vi "CameraServoPWM.vi"(11 "Position":i32) -> ()   [LabVIEW 2018]
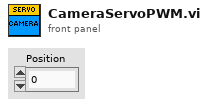
[diagram p1: front panel]
types:
  T1 = typedef "WPI_PWMDeviceRef.ctl" = cluster{"DeviceStatus":errorcluster, "PWM Channel":T2}
  T2 = typedef "FPGA_DIOPWMChannel.ctl" = enum8{"PWM 0", "PWM 1", "PWM 2", "PWM 3", "PWM 4", "PWM 5", "PWM 6", "PWM 7", "PWM 8", "PWM 9", "PWM MXP 0", "PWM MXP 1", "PWM MXP 2", "PWM MXP 3", "PWM MXP 4", "PWM MXP 5", "PWM MXP 6", "PWM MXP 7", "PWM MXP 8", "PWM MXP 9", "Invalid"}
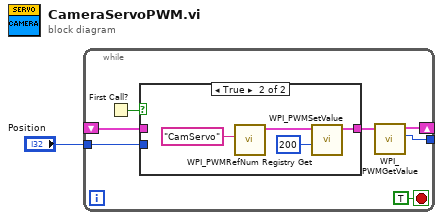
[diagram p0: block diagram]
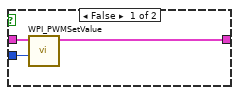
[diagram p2: hidden frame]
diagram:
  n1 = while {
    tunnel: "Position" -> [w8]
    shift-right: [w4] -> _
    shift-left: _ -> [w7]
    tunnel: [w3] -> _
    stop <- TRUE stop-if-true
    n2 = First Call?() -> (First Call?: T/F=w5:bool)
    n3 = case shown="True" w5 {
      tunnel: w8 -> [w10 _]
      tunnel: [w11 w12] -> w2
      tunnel: w7 -> [w9 _]
      frame False {
        n4 = call <vilib>:"WPI_PWMSetValue.vi"("Value"=w10, "PWMDeviceRef"=w9) -> ("PWMDeviceRef"=w11:T1)  [unwired: 8 in, 1 out]
      }
      frame True {
        n5 = call <vilib>:"WPI_PWMRefNum Registry Get.vi"("refnum name"="CamServo") -> ("PWMDeviceRef"=w14:T1)  [unwired: 9 in, 1 out]
        n6 = call <vilib>:"WPI_PWMSetValue.vi"("Value"=200 ("Angle"), "PWMDeviceRef"=w14) -> ("PWMDeviceRef"=w12:T1)  [unwired: 8 in, 1 out]
      }
    }
    n7 = call <vilib>:"WPI_PWMGetValue.vi"("PWMDeviceRef"=w2) -> ("Value"=w3:u16, "PWMDeviceRef"=w4:T1)  [unwired: 8 in, 1 out]
  }
